vi "DDPCA-300.vi"(3 "Gain_Setting":i32(slide)=1 min=1 max=10 step=1 scale=0.5..10.0, 10 "Gain (V/A)":dbl, 11 "Index":i32) -> (2 "Gain (V/A)":dbl)   [LabVIEW 2010]
uses:
  <userlib>/FEMTO/FEMTO_LUCI-10.lvlib
panel:
  in  "Info":bool
  in  "stop":bool
  out "LED":bool
  in  "Check LUCI":bool
  out "String_Product":string
  in  "Product_String":bool
  out "Overload":bool
  in  "Rahmen":bool
  # "Remote Control LUCI-10 DDPCA-300"
  # "Device Information"
  # "DDPCA-300"
  # "Gain Setting"
  # "Overload"
  # "4"
  # "4"
  # "5"
  # "6"
  # "7"
  # "8"
  # "9"
  # "10"
  # "11"
  # "12"
  # "13"
  # "V/A"
  # "10"
  # "10"
  # "10"
  # "10"
  # "10"
  # "10"
  # "10"
  # "10"
  # "10"
  # "10"
  # "10"
  # "10"
  # "10"
  # "10"
  # "10"
  # "10"
  # "10"
  # "10"
  # "10"
  # "10"
  # "Hz"
  # "400"
  # "400"
  # "400"
  # "400"
  # "400"
  # "400"
  # "400"
  # "400"
  # "1"
  # "150"
  # "150"
  # "20"
  # "20"
  # "1"
  # "1"
  # "Sophisticated Tools for Signal Recovery"
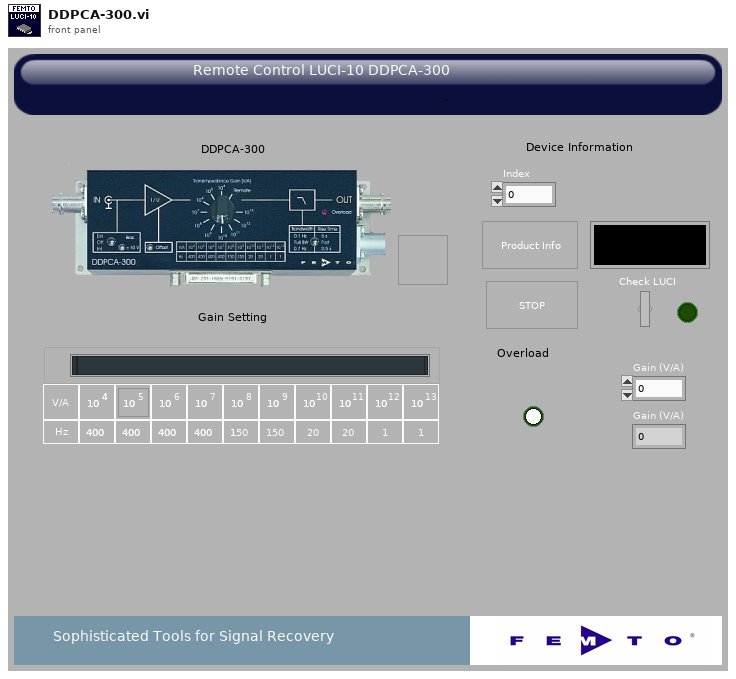
[diagram p1: front panel]
types:
  T1 = enum16{"DDPCA-300", "DLPCA-200", "DHPCA-100", "OE-200", "LIA-MV-150-S", "LIA-MV-150-D", "LIA-MV-200-L", "LIA-MV-200-H", "LIA-MVD-200-L", "LIA-MVD-200-H", "DLPVA-100-BUN-S", "DLPVA-100-BLN-S", "DLPVA-100-B-S", "DLPVA-100-B-D", "DLPVA-100-F-S", "DLPVA-100-F-D", "DHPVA-100", "DHPVA-200", "DUPVA-1-60", "DUPVA-1-70"}
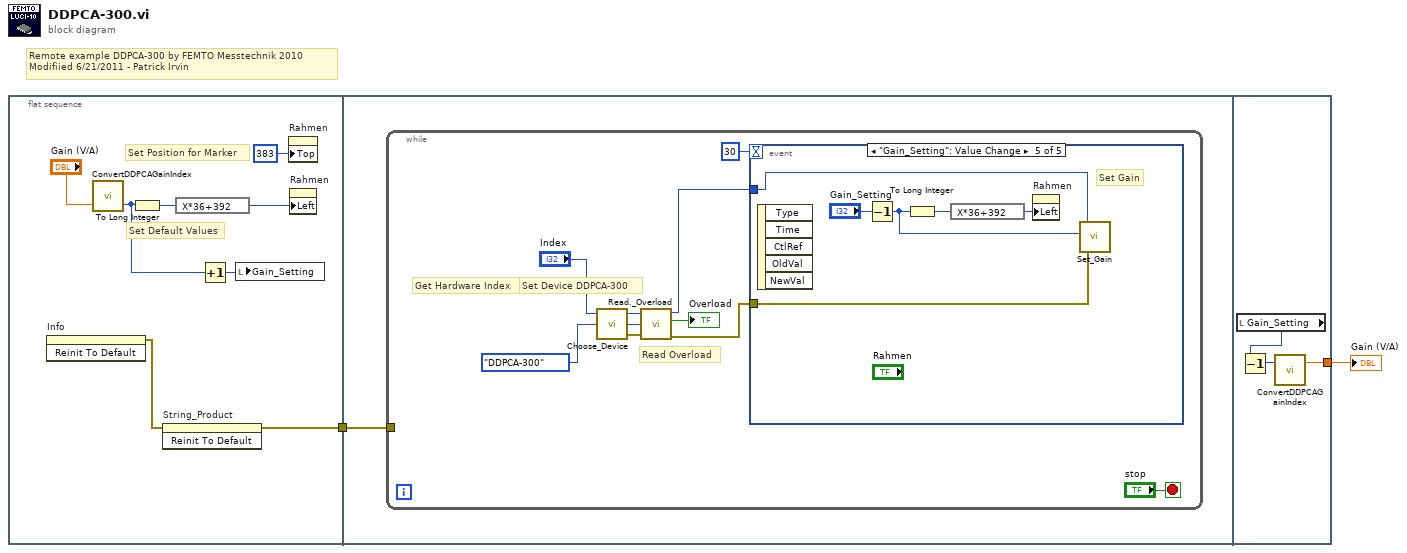
[diagram p0: block diagram]
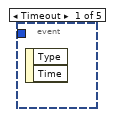
[diagram p2: hidden frame]
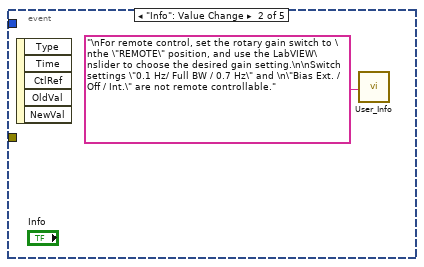
[diagram p3: hidden frame]
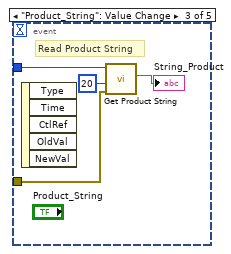
[diagram p4: hidden frame]
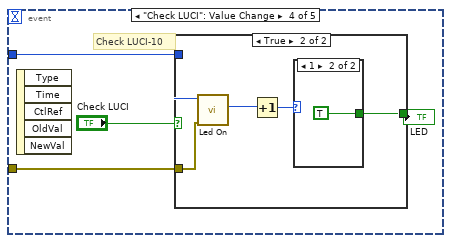
[diagram p5: hidden frame]
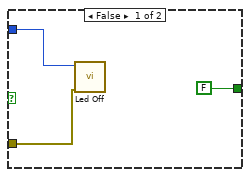
[diagram p6: hidden frame]
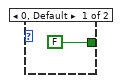
[diagram p7: hidden frame]
diagram:
  # "Remote example DDPCA-300 by FEMTO Messtechnik 2010\nModifiied 6/21/2011 - Patrick Irvin"
  n1 = flat-sequence {
    tunnel: [w6] -> w2
    tunnel: w2 -> [w11]
    tunnel: [w47] -> w1
    frame #0 {
      # "Set Default Values"
      # "Set Position for Marker"
      n2 = invoke on="Info" class="Bool" method="Reinit To Default"() -> (error out=w7:errorcluster)  [unwired: 3 in, 2 out]
      n3 = call "ConvertDDPCAGainIndex.vi"("Gain (V/A)"="Gain (V/A)") -> ("Gain (Index)"=w3:i32)  [unwired: 1 in, 1 out]
      n4 = To Long Integer(number=w3) -> (32bit integer=w9:i32)
      n5 = invoke on="String_Product" class="Str" method="Reinit To Default"(error in=w7) -> (error out=w6:errorcluster)  [unwired: 2 in, 2 out]
      n6 = expression code="X*36+392"(w9) -> (w10:i32)
      n7 = Increment(x=w3) -> (x+1=w4:i32)
      n8 = local write "Gain_Setting"(w4) -> ()
      n9 = property on="Rahmen" class="Bool"("Top"=383 ("Position:Top")) -> ()  [unwired: 2 in, 2 out]
      n10 = property on="Rahmen" class="Bool"("Left"=w10) -> ()  [unwired: 2 in, 2 out]
    }
    frame #1 {
      n11 = while {
        tunnel: w11 -> [_]
        stop <- "stop" stop-if-true
        # "Get Hardware Index"
        # "Read Overload"
        # "Set Device DDPCA-300"
        n12 = call <userlib>:"Choose_Device.vi"("Choose_Device"=T1."DDPCA-300", "Index"="Index") -> ("error out"=w20:errorcluster, "Device_type"=w19:T1, "Index_Out"=w18:i32)  [unwired: 1 in]
        n13 = call <userlib>:"Read._Overload.vi"("Index"=w18, "Choose_Device"=w19, "error in (no error)"=w20) -> ("Index_Out"=w15:i32, "Overload"=→"Overload":bool, "error out"=w14:errorcluster)  [unwired: 1 out]
        n14 = event shown="[4] \"Gain_Setting\": Value Change" {
          selector: _ -> [_ _ _ _ _]
          dyn-events: _ -> [_ _ _ _ _]
          timeout: 30 -> [_ _ _ _ _]
          tunnel: w15 -> [_ _ w26 w30 w44]
          tunnel: w14 -> [_ _ w24 w29 w43]
          event Timeout {
            n15 = event-data() -> ()  [unwired: 3 out]
          }
          event "Info": Value Change {
            n16 = event-data() -> ()  [unwired: 6 out]
            n17 = call <userlib>:"User_Info.vi"("String"="\nFor remote control, set the rotary gain switch to \nthe \"REMOTE\" position, and use the LabVIEW\nslider to choose the desired gain setting.\n\nSwitch settings \"0.1 Hz/ Full BW / 0.7 Hz\" and \n\"Bias Ext. / Off / Int.\" are not remote controllable.") -> ()  [unwired: 1 out]
          }
          event "Product_String": Value Change {
            # "Read Product String"
            n18 = event-data() -> ()  [unwired: 6 out]
            n19 = call <userlib>:"Get Product String.vi"("error in (no error)"=w24, "size"=20, "index"=w26) -> ("string out"=→"String_Product":string)  [unwired: 8 out]
          }
          event "Check LUCI": Value Change {
            # "Check LUCI-10"
            n20 = event-data() -> ()  [unwired: 6 out]
            n21 = case shown="True" "Check LUCI" {
              tunnel: w30 -> [w33 w38]
              tunnel: w29 -> [w32 w37]
              tunnel: [FALSE w34] -> w27
              frame False {
                n22 = call <userlib>:"Led Off.vi"("error in (no error)"=w32, "index"=w33) -> ()  [unwired: 10 out]
              }
              frame True {
                n23 = call <userlib>:"Led On.vi"("error in (no error)"=w37, "index"=w38) -> ("function_return"=w36:i32)  [unwired: 9 out]
                n24 = Increment(x=w36) -> (x+1=w35:i32)
                n25 = case shown="1" w35 {
                  tunnel: [FALSE TRUE] -> w34
                  frame 0, Default {
                  }
                  frame 1 {
                  }
                }
              }
            }
            "LED" <- w27
          }
          event "Gain_Setting": Value Change {
            # "Set Gain"
            n26 = event-data() -> ()  [unwired: 6 out]
            n27 = Decrement(x="Gain_Setting") -> (x-1=w41:i32)
            n28 = To Long Integer(number=w41) -> (32bit integer=w46:i32)
            n29 = expression code="X*36+392"(w46) -> (w42:i32)
            n30 = property on="Rahmen" class="Bool"("Left"=w42) -> ()  [unwired: 2 in, 2 out]
            n31 = call-poly <userlib>:"Set_Gain.vi"("error in"=w43, "Gain [V/A]"=w41, "index"=w44) -> ()  [unwired: 1 in, 3 out]
          }
        }
      }
    }
    frame #2 {
      n32 = local read "Gain_Setting"() -> (w49:i32)
      n33 = Decrement(x=w49) -> (x-1=w48:i32)
      n34 = call "ConvertDDPCAGainIndex.vi"("Gain (Index)"=w48) -> ("Gain (V/A)"=w47:dbl)  [unwired: 1 in, 1 out]
    }
  }
  "Gain (V/A)" <- w1
